vi "Get JSON CFG.vi"(11 "CFG Base in":refnum<class "CFG Base.lvclass">) -> (2 "<JSON>CFG":string, 3 "CFG Base out":refnum<class "CFG Base.lvclass">)   [LabVIEW 2024, in "HAL.lvlib" / "CFG Base.lvclass"]
uses:
  CFG Base.lvclass
  CFG Base.lvclass/CFG Base.ctl
  <vilib>/JDP Science/JSONtext/Config Files/Config File.lvclass/Config File.ctl
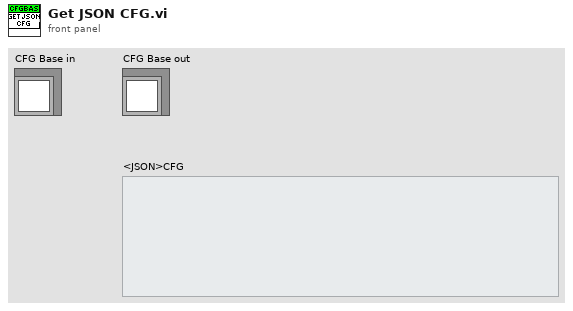
[diagram p1: front panel]
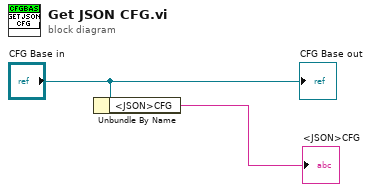
[diagram p0: block diagram]
diagram:
  n1 = Unbundle By Name("CFG Base in") -> ("<JSON>CFG"=→"<JSON>CFG":string)
  "CFG Base out" <- "CFG Base in"
